vi "Global.vi"() -> ()   [LabVIEW 2014]
panel:
  out "Video Stream 2":picture
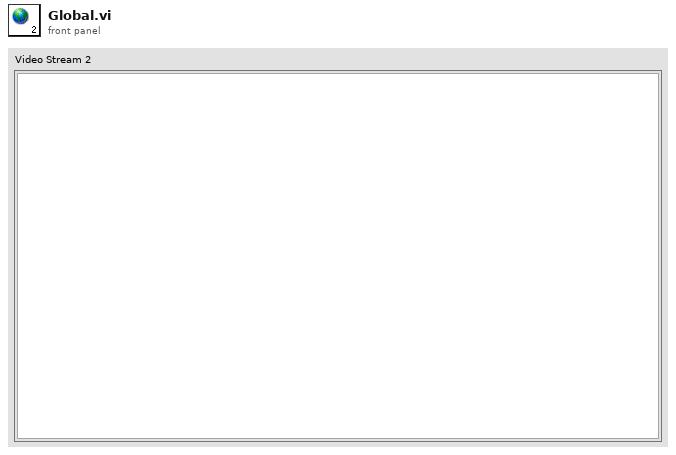
[diagram p1: front panel]
diagram:
